vi "VITester_Item_Init.vi"(11 "Object":T1) -> ()   [LabVIEW 2009]
uses:
  Support/VITester Project Item Ref.ctl
  API/mxLvMenuItem.ctl
panel:
  out "error out":errorcluster
  in  "error in":errorcluster
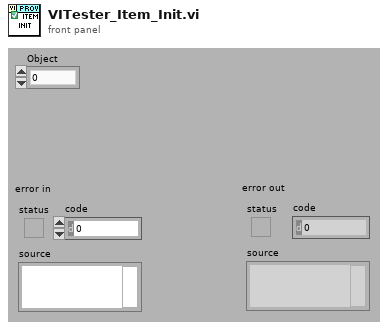
[diagram p1: front panel]
types:
  T1 = typedef "VITester Project Item Ref.ctl" = u64
  T2 = typedef "mxLvMenuItem.ctl" = cluster{"Menu Name":string, "Description":string, "Icon File Name":path, "Menu Tag":string, "Enabled":bool, "Checked":bool, "Separator":bool, "Batchable":bool, "Weight":i32, "Batch Mode (Ignored if Not Batchable)":enum32{"Show If All Items Support Command", "Show If Any Items Support Command"}, "Menu Location":enum32{"<None>", "Project", "Project / Build Specifications", "Tools", "Tools / Source Control", "Tools / Real-Time Module", "Help"}, "Exclude From Getting Started Window Menu":bool}
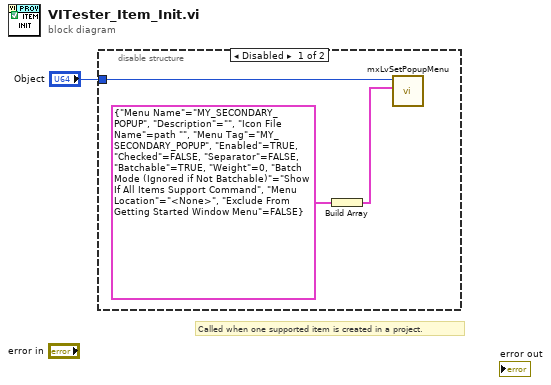
[diagram p0: block diagram]
diagram:
  # "Called when one supported item is created in a project."
  n1 = disable-structure shown="Disabled" {
    disable-tunnel: "Object" -> [w4 _]
    frame #0 {
      n2 = Build Array(T2 {"Menu Name"="MY_SECONDARY_POPUP", "Description"="", "Icon File Name"=path "", "Menu Tag"="MY_SECONDARY_POPUP", "Enabled"=TRUE, "Checked"=FALSE, "Separator"=FALSE, "Batchable"=TRUE, "Weight"=0, "Batch Mode (Ignored if Not Batchable)"=enum."Show If All Items Support Command", "Menu Location"=enum."<None>", "Exclude From Getting Started Window Menu"=FALSE} ("Menu Item")) -> (w3:T2[])
      n3 = call "mxLvSetPopupMenu.vi"("Popup Menu Items"=w3, "Item"=w4) -> ()  [unwired: 8 in, 2 out]
    }
    frame #1 {
    }
  }
